vi "zadanie 2.vi"() -> ()   [LabVIEW 2013]
panel:
  out "Массив В":dbl[][](array[numeric])
  out "Массив А":dbl[][](array[numeric])
  out "Вывод":dbl[][](array[numeric])
  in  "Numeric":dbl
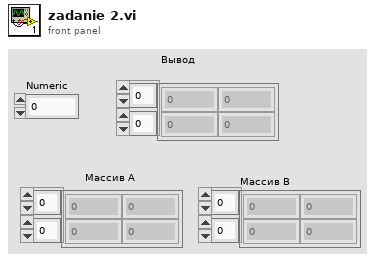
[diagram p1: front panel]
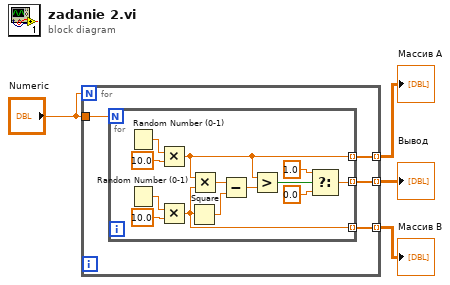
[diagram p0: block diagram]
diagram:
  n1 = for {
    N: "Numeric" -> [_]
    tunnel: "Numeric" -> [w8]
    tunnel: [w7] -> w3 mode=indexing
    tunnel: [w6] -> w2 mode=indexing
    tunnel: [w5] -> w1 mode=indexing
    n2 = for {
      N: w8 -> [_]
      tunnel: [w15] -> w7 mode=indexing
      tunnel: [w10] -> w6 mode=indexing
      tunnel: [w9] -> w5 mode=indexing
      n3 = Random Number (0-1)() -> (number: 0 to 1=w14:dbl)
      n4 = Random Number (0-1)() -> (number: 0 to 1=w12:dbl)
      n5 = Multiply(x=w14, y=10.0) -> (x*y=w10:dbl)
      n6 = Multiply(x=w12, y=10.0) -> (x*y=w9:dbl)
      n7 = Square(x=w9) -> (x^2=w19:dbl)
      n8 = Multiply(x=w10, y=w9) -> (x*y=w18:dbl)
      n9 = Subtract(x=w18, y=w19) -> (x-y=w17:dbl)
      n10 = Greater?(x=w10, y=w17) -> (0:w16:bool)
      n11 = Select(t=1.0, s=w16, f=0.0) -> (s? t:f=w15:dbl)
    }
  }
  "Вывод" <- w3
  "Массив А" <- w2
  "Массив В" <- w1
